vi "CRYSet Units setup Front Panel.vi"(11 "Vi Ref":refnum<vi>) -> ()   [LabVIEW 2013]
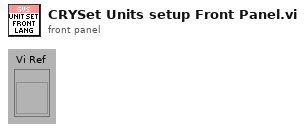
[diagram p1: front panel]
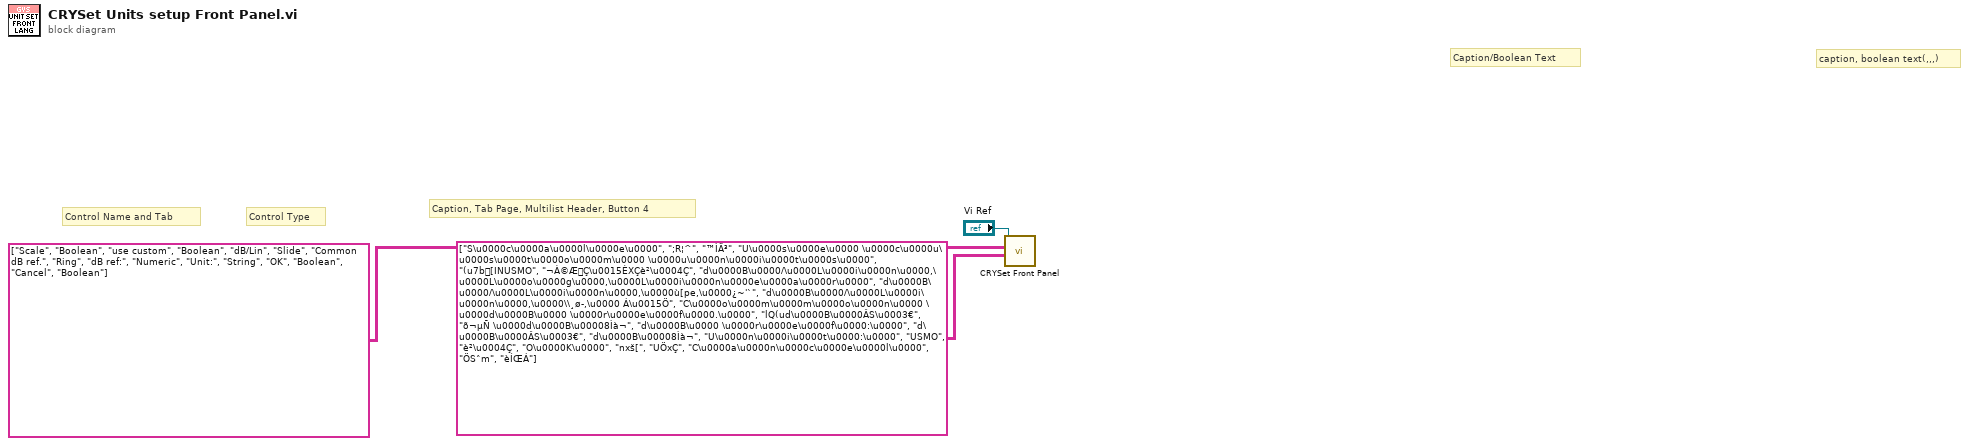
[diagram p0: block diagram]
diagram:
  # "Caption, Tab Page, Multilist Header, Button 4"
  # "Control Type"
  # "Control Name and Tab"
  # "caption, boolean text(,,,)"
  # "Caption/Boolean Text"
  n1 = call "CRYSet Front Panel.vi"("Caption(Boolean Text)"=string[][] [["S\u0000c\u0000a\u0000l\u0000e\u0000", ";R¦^", "™ÌÄ³"], ["U\u0000s\u0000e\u0000 \u0000c\u0000u\u0000s\u0000t\u0000o\u0000m\u0000 \u0000u\u0000n\u0000i\u0000t\u0000s\u0000", "(u7bꁚ[INUSMO", "¬À©ÆÇ\u0015ÈXÇè²\u0004Ç"], ["d\u0000B\u0000/\u0000L\u0000i\u0000n\u0000,\u0000L\u0000o\u0000g\u0000,\u0000L\u0000i\u0000n\u0000e\u0000a\u0000r\u0000", "d\u0000B\u0000/\u0000L\u0000i\u0000n\u0000,\u0000ù[pe,\u0000¿~'`", "d\u0000B\u0000/\u0000L\u0000i\u0000n\u0000,\u0000\\¸ø­,\u0000 Á\u0015Ö"], ["C\u0000o\u0000m\u0000m\u0000o\u0000n\u0000 \u0000d\u0000B\u0000 \u0000r\u0000e\u0000f\u0000.\u0000", "lQ(ud\u0000B\u0000ÂS\u0003€", "õ¬µÑ \u0000d\u0000B\u00008Ìà¬"], ["d\u0000B\u0000 \u0000r\u0000e\u0000f\u0000:\u0000", "d\u0000B\u0000ÂS\u0003€", "d\u0000B\u00008Ìà¬"], ["U\u0000n\u0000i\u0000t\u0000:\u0000", "USMO", "è²\u0004Ç"], ["O\u0000K\u0000", "nxš[", "UÖxÇ"], ["C\u0000a\u0000n\u0000c\u0000e\u0000l\u0000", "ÖSˆm", "èÍŒÁ"]], "Control ID and Type(Label Name, Type)"=string[][] [["Scale", "Boolean"], ["use custom", "Boolean"], ["dB/Lin", "Slide"], ["Common dB ref.", "Ring"], ["dB ref:", "Numeric"], ["Unit:", "String"], ["OK", "Boolean"], ["Cancel", "Boolean"]], "Vi Ref"="Vi Ref") -> ()  [unwired: 9 in]
